vi "Delete Control from Cluster.vi"(8 "error in (no error)":errorcluster, 10 "Control Name in":string, 11 "Cluster ref in":refnum<vi>) -> (0 "error out":errorcluster, 2 "Deleted Index":i32, 3 "Cluster ref out":refnum<vi>)   [LabVIEW 2019, in "gRPC Scripting Tools.lvlib"]
uses:
  gRPC Scripting Tools.lvlib
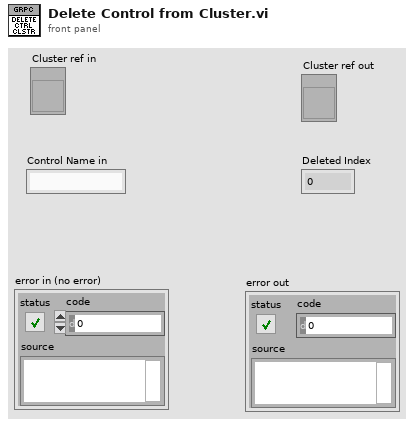
[diagram p1: front panel]
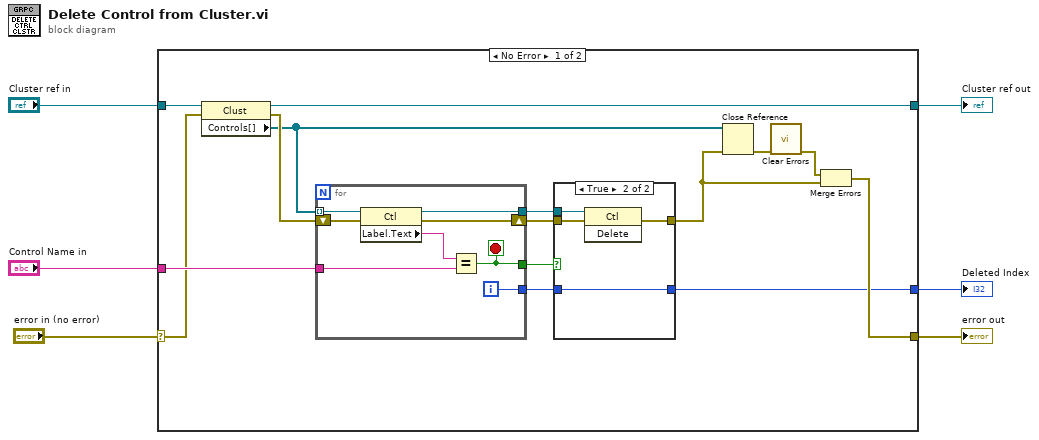
[diagram p0: block diagram]
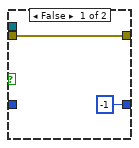
[diagram p2: hidden frame]
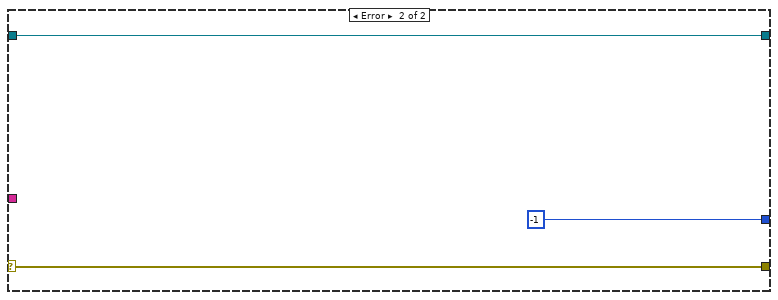
[diagram p3: hidden frame]
diagram:
  n1 = case shown="No Error" "error in (no error)" {
    selector: "error in (no error)" -> [w10 w38]
    tunnel: "Control Name in" -> [w21 _]
    tunnel: [w20 w38] -> w5
    tunnel: [w16 w37] -> w4
    tunnel: "Cluster ref in" -> [w11 w37]
    tunnel: [w7 -1] -> w1
    frame No Error {
      n2 = property class="Clust"(reference=w11, error in=w10) -> (reference out=w16:refnum<vi>, error out=w14:errorcluster, "Controls[]"=w13:refnum<vi>[])
      n3 = for {
        tunnel: w21 -> [w35]
        tunnel: w13 -> [w34] mode=indexing
        tunnel: [w33] -> w12
        tunnel: [w32] -> w8
        shift-right: [w29] -> w15
        shift-left: w14 -> [w30]
        tunnel: [w28] -> w9
        i -> [w32]
        stop <- w28 stop-if-true
        n4 = property class="Ctl"(reference=w34, error in=w30) -> (reference out=w33:refnum<vi>, error out=w29:errorcluster, "Label.Text"=w31:string)
        n5 = Equal?(x=w31, y=w35) -> (x = y?=w28:bool)
      }
      n6 = case shown="True" w9 {
        tunnel: [w23 w27] -> w18
        tunnel: w15 -> [w23 w26]
        tunnel: w12 -> [_ w25]
        tunnel: w8 -> [_ w24]
        tunnel: [-1 w24] -> w7
        frame False {
        }
        frame True {
          n7 = invoke class="Ctl" method="Delete"(reference=w25, error in=w26) -> (error out=w27:errorcluster)  [unwired: 1 in, 2 out]
        }
      }
      n8 = Close Reference(reference=w13, error in (no error)=w18) -> (error out=w17:errorcluster)
      n9 = call <vilib>:"Clear Errors.vi"("error in (no error)"=w17) -> ("error out"=w19:errorcluster)  [unwired: 5 in, 1 out]
      n10 = Merge Errors(w19, w18) -> (w20:errorcluster)
    }
    frame Error {
    }
  }
  "error out" <- w5
  "Cluster ref out" <- w4
  "Deleted Index" <- w1
